vi "normalize.vi"(9 "index2":dbl, 10 "index1":dbl, 11 "index0":dbl) -> (0 "index2":dbl, 1 "index1":dbl, 2 "index0":dbl, 3 "Array Output":dbl[](array[numeric]))   [LabVIEW 2017]
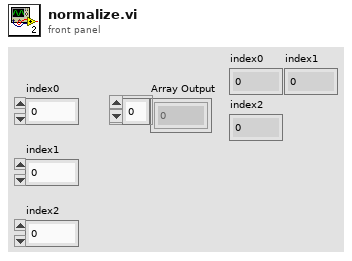
[diagram p1: front panel]
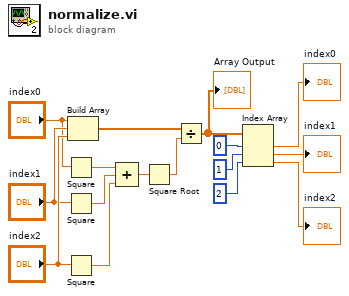
[diagram p0: block diagram]
diagram:
  n1 = Square(x="index0") -> (x^2=w13:dbl)
  n2 = Square(x="index1") -> (x^2=w14:dbl)
  n3 = Square(x="index2") -> (x^2=w15:dbl)
  n4 = Build Array("index0", "index1", "index2") -> (w16:dbl[])
  n5 = Compound Arithmetic op=ADD(w13, w14, w15) -> (w2:dbl)
  n6 = Square Root(x=w2) -> (sqrt(x)=w1:dbl)
  n7 = Divide(x=w16, y=w1) -> (x/y=w9:dbl[])
  "Array Output" <- w9
  n8 = Index Array(array=w9, index #1=0 ("index"), index #2=1 ("index"), index #3=2 ("index")) -> (element #1=→"index0":dbl, element #2=→"index1":dbl, element #3=→"index2":dbl)
